vi "CoMP-S Mechanism - Rotation Verification2.vi"(8 "error in (no error)":errorcluster, 10 "Motors":bool, 11 "Rotation":dbl format="%.1f") -> (0 "error out":errorcluster, 3 "Rotation out":dbl format="%#.1f")   [LabVIEW 2014]
panel:
  out "String 2":string
  in  "OK":bool
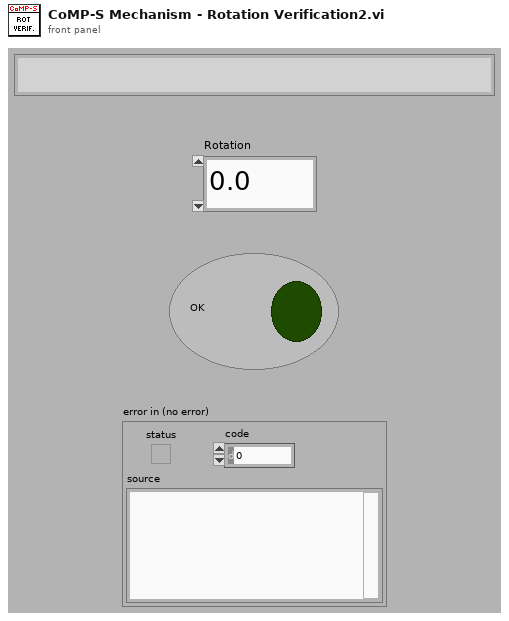
[diagram p1: front panel]
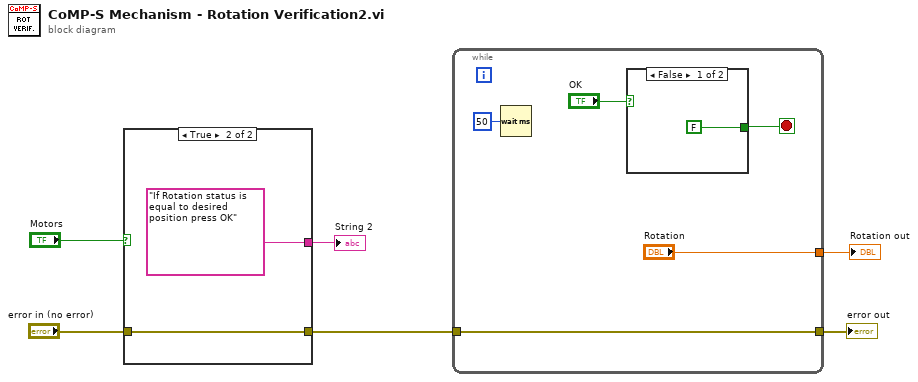
[diagram p0: block diagram]
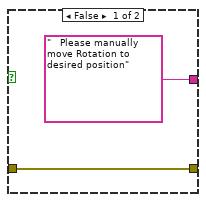
[diagram p2: hidden frame]
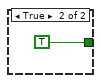
[diagram p3: hidden frame]
diagram:
  n1 = case shown="True" "Motors" {
    tunnel: ["   Please manually move Rotation to desired position" ("String") "If Rotation status is equal to desired position press OK" ("String")] -> w4
    tunnel: [w8 w9] -> w5
    tunnel: "error in (no error)" -> [w8 w9]
    frame False {
    }
    frame True {
    }
  }
  "String 2" <- w4
  n2 = while {
    tunnel: w5 -> [w12]
    tunnel: [w12] -> w6
    tunnel: ["Rotation"] -> w1
    stop <- w13 stop-if-true
    n3 = Wait (ms)(milliseconds to wait=u32 50) -> ()  [unwired: 1 out]
    n4 = case shown="False" "OK" {
      tunnel: [FALSE TRUE] -> w13
      frame False {
      }
      frame True {
      }
    }
  }
  "error out" <- w6
  "Rotation out" <- w1
